vi "sub_extrace_bonding_wf.vi"(10 "Bonding force":dbl, 11 "Trigger graph":waveform(dbl)(graph)) -> (2 "b_info":T1, 3 "Bonding":waveform(dbl)(graph) caption="Bonding_wf")   [LabVIEW 2016]
uses:
  <vilib>/Analysis/baseanly.llb/Mean (DBL).vi
  <vilib>/Waveform/WDTOps.llb/WDT Waveform Duration DBL.vi
  <vilib>/measure/mamon.llb/Trigger Detection for 1 Channel.vi
  <vilib>/Waveform/WDTOps.llb/WDT Get Waveform Subset DBL.vi
  <vilib>/Analysis/baseanly.llb/Unimode.vi
  Global.vi
  <vilib>/measure/NI_MAPro.lvlib
  <vilib>/Analysis/NI_AALBase.lvlib
panel:
  out "standard deviation":dbl caption="표준편차" format="%0.2f"
  out "웨이브폼 차트 2":cluster{"mode":dbl, "mean":dbl}(graph)
  out "bonding f":dbl
  out "mean":dbl caption="평균" format="%0.2f"
  out "웨이브폼 그래프":dbl[](graph)
  out "웨이브폼 차트":cluster{"mean":dbl, dbl}(graph)
  out "rising_index":dbl
  out "falling_index":dbl
  out "trigger_B_rising":dbl format="%#_2g"
  out "trigger_B_falling":dbl format="%#_2g"
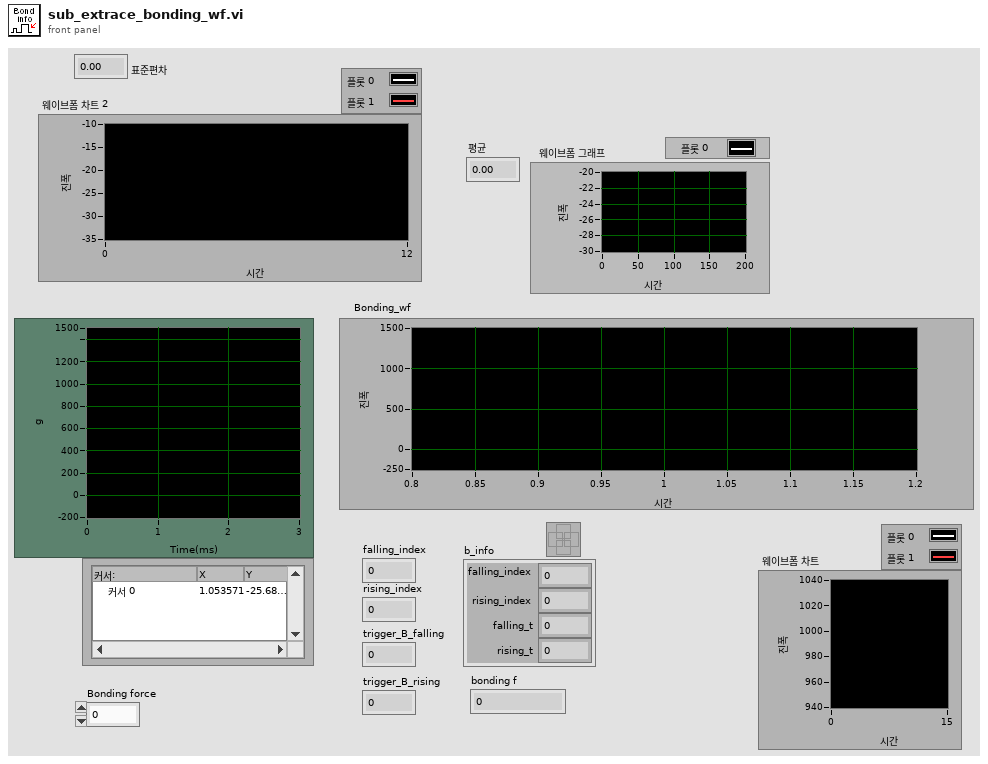
[diagram p1: front panel]
types:
  T1 = cluster{"falling_index":dbl, "rising_index":dbl, "falling_t":dbl, "rising_t":dbl}
  T2 = typedef "data.ctl" = cluster{"Bonding force":dbl, "Bonding time":dbl, "Bonding index":dbl, "Pickup force":dbl, "Pickup time":dbl, "Pickup index":dbl, "Detach force":dbl, "Detach time":dbl, "Detach index":dbl, "Heater temp rt":dbl, "Vacuum rt":dbl, "IR raw data":i16[][], "IR temp data":dbl[][], "vacuum raw wf":waveform(dbl), "vacuum kpa wf":waveform(dbl), "strain raw wf":waveform(dbl)[], "Force rt":dbl, "Vacuum T":dbl, "Heater temp T":dbl, "Balance xy arrays":cluster{dbl, dbl}[], "Balance xy":cluster{dbl, dbl}[], "Bonding wf index":dbl, "Pickup wf index":dbl, "Bonding rising index":dbl, "Bonding falling index":dbl, "Pickup rising index":dbl, "Pickup falling index":dbl}
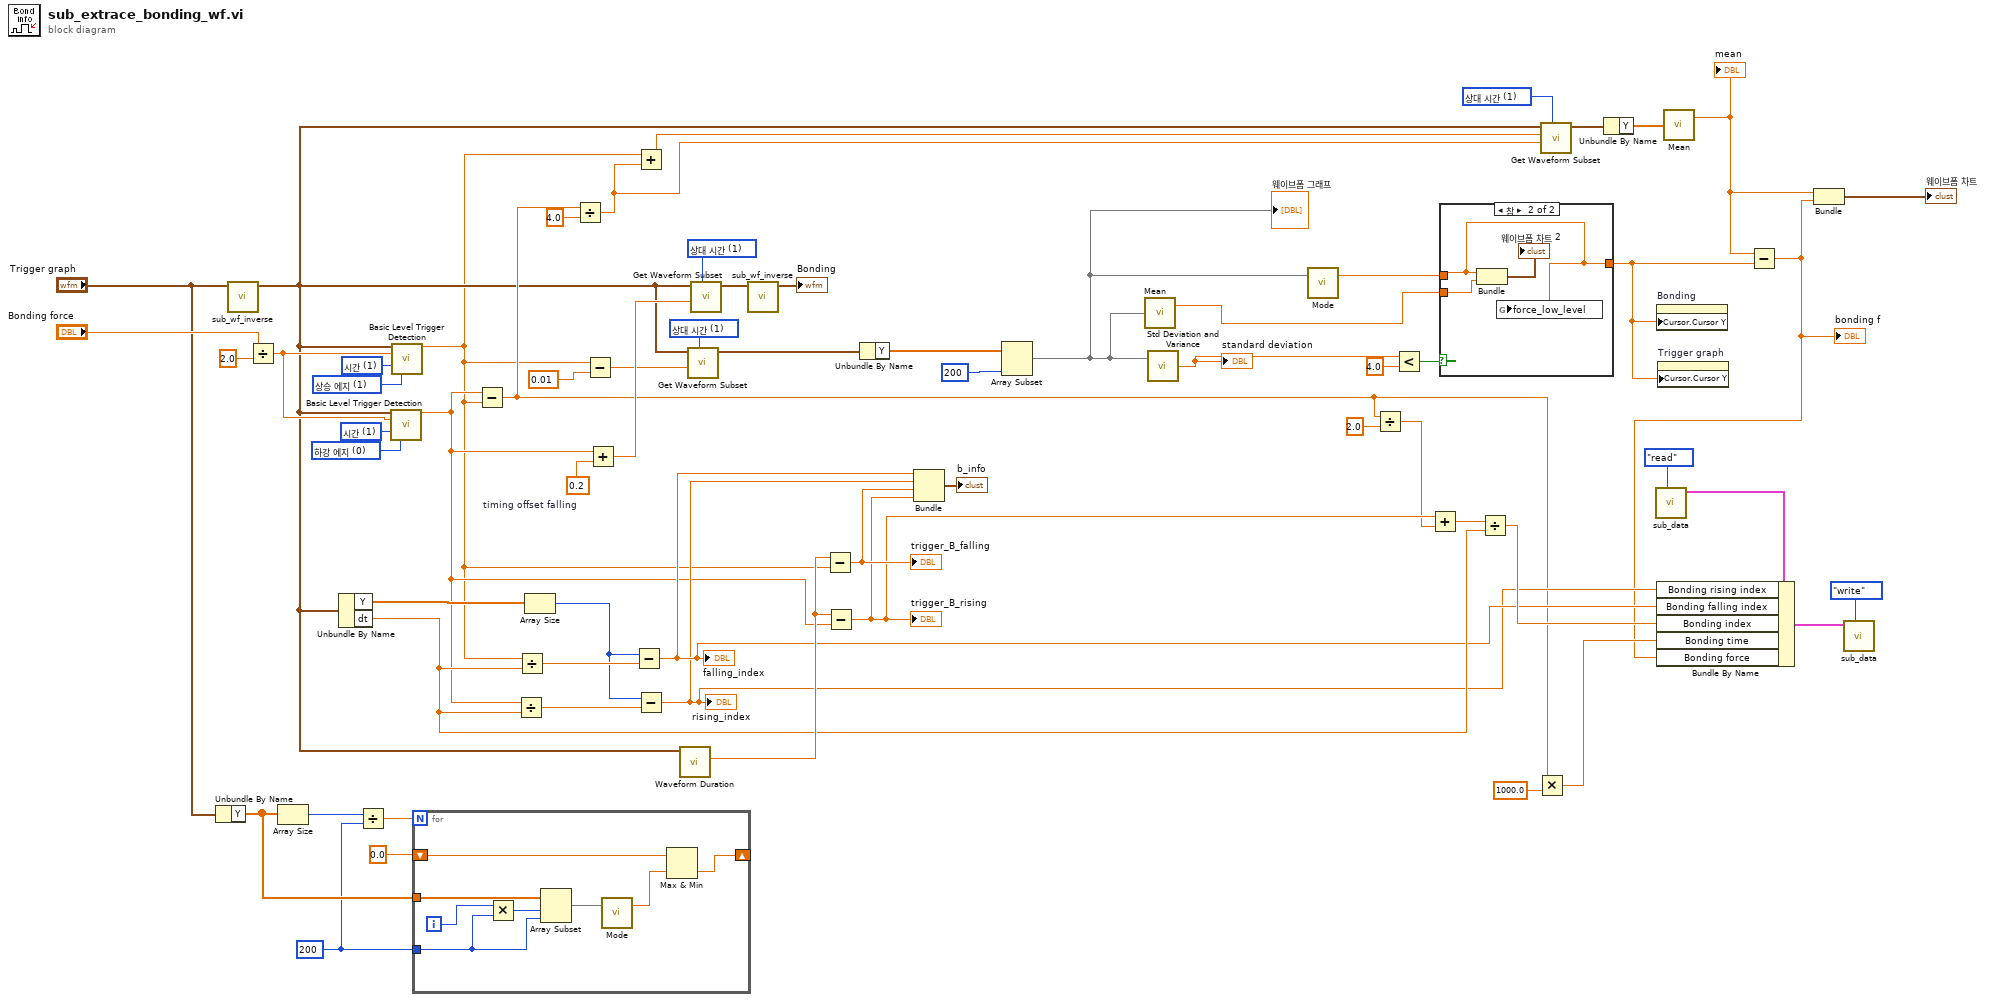
[diagram p0: block diagram]
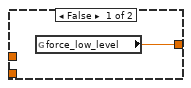
[diagram p2: hidden frame]
diagram:
  w14 = u16 1 items=["샘플 ", "상대 시간"] ("start/duration format")
  w25 = u16 1 items=["샘플 ", "상대 시간"] ("start/duration format")
  w29 = 200 ("block size")
  w57 = 0.2  # timing offset falling
  w60 = u16 1 items=["샘플 ", "상대 시간"] ("start/duration format")
  w61 = u16 0 items=["하강 에지", "상승 에지"] ("trigger slope")
  w62 = u16 1 items=["인덱스", "시간"] ("location mode")
  w63 = u16 1 items=["하강 에지", "상승 에지"] ("trigger slope")
  w64 = u16 1 items=["인덱스", "시간"] ("location mode")
  n1 = Unbundle By Name("Trigger graph") -> ("Y"=w32:dbl[])
  n2 = call "sub_wf_inverse.vi"("Trigger graph"="Trigger graph") -> ("inverse graph"=w15:waveform(dbl))  [unwired: 10 in]
  n3 = Divide(x="Bonding force", y=2.0) -> (x/y=w58:dbl)
  n4 = Array Size(array=w32) -> (size(s)=w31:i32)
  n5 = Unbundle By Name(w15) -> ("Y"=w54:dbl[], "dt"=w41:dbl)
  n6 = Divide(x=w31, y=w29) -> (x/y=w34:dbl)
  n7 = call-poly <vilib>:"Basic Level Trigger Detection.vi"("signal in"=w15, "level"=w58, "location mode"=w62, "trigger slope"=w61) -> ("trigger location"=w30:dbl)  [unwired: 9 in, 2 out]
  n8 = call-poly <vilib>:"Basic Level Trigger Detection.vi"("signal in"=w15, "level"=w58, "location mode"=w64, "trigger slope"=w63) -> ("trigger location"=w13:dbl)  [unwired: 9 in, 2 out]
  n9 = for {
    N: w34 -> [_]
    tunnel: w32 -> [w73]
    shift-right: [w67] -> _
    shift-left: 0.0 ("y") -> [w68]
    tunnel: w29 -> [w66]
    i -> [w71]
    n10 = Multiply(x=w71, y=w66) -> (x*y=w72:i32)
    n11 = Array Subset(array=w73, index=w72, length=w66) -> (w70:dbl[])
    n12 = call-poly <vilib>:"Mode.vi"("X"=w70) -> ("mode"=w69:dbl)  [unwired: 1 in, 1 out]
    n13 = Max & Min(x=w68, y=w69) -> (min(x,y)=w67:dbl)  [unwired: 1 out]
  }
  n14 = Subtract(x=w30, y=w13) -> (x-y=w23:dbl)
  n15 = Divide(x=w30, y=w41) -> (x/y=w50:dbl)
  n16 = Divide(x=w13, y=w41) -> (x/y=w53:dbl)
  n17 = Array Size(array=w54) -> (size(s)=w51:i32)
  n18 = Divide(x=w23, y=4.0) -> (x/y=w21:dbl)
  n19 = Subtract(x=w13, y=0.01 ("y 2")) -> (x-y=w11:dbl)
  n20 = Add(x=w30, y=w57) -> (x+y=w59:dbl)
  n21 = Subtract(x=w51, y=w53) -> (x-y=w38:dbl)
  "falling_index" <- w38
  n22 = Add(x=w13, y=w21) -> (x+y=w22:dbl)
  n23 = Subtract(x=w51, y=w50) -> (x-y=w37:dbl)
  "rising_index" <- w37
  n24 = call-poly <vilib>:"Waveform Duration.vi"("waveform in"=w15) -> ("duration"=w52:dbl)  [unwired: 8 in, 2 out]
  n25 = call-poly <vilib>:"Get Waveform Subset.vi"("start/duration format"=w14, "duration"=w11, "waveform in"=w15) -> ("waveform out"=w5:waveform(dbl))  [unwired: 3 in, 3 out]
  n26 = call-poly <vilib>:"Get Waveform Subset.vi"("start/duration format"=w60, "duration"=w59, "waveform in"=w15) -> ("waveform out"=w55:waveform(dbl))  [unwired: 3 in, 3 out]
  n27 = call "sub_wf_inverse.vi"("Trigger graph"=w55) -> ("inverse graph"=→"Bonding":waveform(dbl))  [unwired: 10 in]
  n28 = Subtract(x=w52, y=w13) -> (x-y=w43:dbl)
  "trigger_B_falling" <- w43
  n29 = Subtract(x=w52, y=w30) -> (x-y=w36:dbl)
  "trigger_B_rising" <- w36
  n30 = Unbundle By Name(w5) -> ("Y"=w4:dbl[])
  n31 = Bundle(w38, w37, w43, w36) -> (→"b_info":cluster{dbl, dbl, dbl, dbl})  [unwired: 1 in]
  n32 = Array Subset(array=w4, length=200 ("길이")) -> (w2:dbl[])  [unwired: 1 in]
  "웨이브폼 그래프" <- w2
  n33 = call-poly <vilib>:"Mean.vi"("X"=w2) -> ("mean"=w7:dbl)  [unwired: 1 out]
  n34 = call <vilib>:"Std Deviation and Variance.vi"("X"=w2) -> ("standard deviation"=w9:dbl)  [unwired: 1 in, 2 out]
  "standard deviation" <- w9
  n35 = call-poly <vilib>:"Mode.vi"("X"=w2) -> ("mode"=w6:dbl)  [unwired: 1 in, 1 out]
  n36 = Divide(x=w23, y=2.0) -> (x/y=w26:dbl)
  n37 = Less?(x=w9, y=4.0) -> (x < y?=w8:bool)
  n38 = Add(x=w36, y=w26) -> (x+y=w42:dbl)
  n39 = case shown="참" w8 {
    tunnel: w7 -> [_ w77]
    tunnel: w6 -> [_ w75]
    tunnel: [w74 w75] -> w1
    frame False {
      n40 = global read "Global.vi" "force_low_level"() -> (w74:dbl)
    }
    frame True {
      n41 = Bundle("mode"=w75, "mean"=w77) -> (→"웨이브폼 차트 2":cluster{"mode":dbl, "mean":dbl})  [unwired: 1 in]
      n42 = global write "Global.vi" "force_low_level"(w75) -> ()
    }
  }
  n43 = Divide(x=w42, y=w41) -> (x/y=w39:dbl)
  n44 = Multiply(x=w23, y=1000.0) -> (x*y=w44:dbl)
  n45 = call-poly <vilib>:"Get Waveform Subset.vi"("start/duration format"=w25, "duration"=w21, "start samples/time"=w22, "waveform in"=w15) -> ("waveform out"=w20:waveform(dbl))  [unwired: 2 in, 3 out]
  n46 = Unbundle By Name(w20) -> ("Y"=w19:dbl[])
  n47 = call "sub_data.vi"("cmd"=enum16{"ini", "write", "read"}."read") -> ("data out"=w46:T2)  [unwired: 9 in, 1 out]
  n48 = property on="Bonding" class="WFGraph (엄격한)"("Cursor.Cursor Y"=w1) -> ()  [unwired: 2 in, 2 out]
  n49 = property on="Trigger graph" class="WFGraph (엄격한)"("Cursor.Cursor Y"=w1) -> ()  [unwired: 2 in, 2 out]
  n50 = call-poly <vilib>:"Mean.vi"("X"=w19) -> ("mean"=w18:dbl)  [unwired: 1 out]
  "mean" <- w18
  n51 = Subtract(x=w18, y=w1) -> (x-y=w16:dbl)
  "bonding f" <- w16
  n52 = Bundle By Name(cluster=w46, "Bonding rising index"=w37, "Bonding falling index"=w38, "Bonding index"=w39, "Bonding time"=w44, "Bonding force"=w16) -> (w49:T2)
  n53 = Bundle("mean"=w18, w16) -> (→"웨이브폼 차트":cluster{"mean":dbl, dbl})  [unwired: 1 in]
  n54 = call "sub_data.vi"("cmd"=enum16{"ini", "write", "read"}."write", "data in"=w49) -> ()  [unwired: 8 in, 2 out]
